vi "ROS_Topic_Close.vi"(0 "error in":errorcluster, 2 "topic":string, 3 "StopConsole":bool=TRUE) -> (1 "error out":errorcluster)   [LabVIEW 2012]
doc: "Closes a topic. If no topic is defined, it will close all tasks and close the console (unless specified otherwise)."
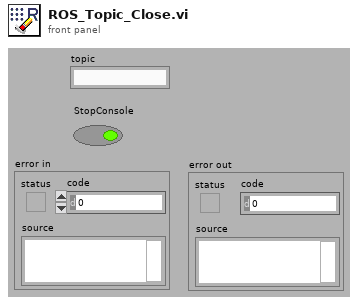
[diagram p1: front panel]
types:
  T1 = enum16{"Add Server", "Clear Server", "Clear All", "Get Info"}
  T2 = typedef "ServoInfo.ctl" = cluster{"vi name":string, "VI Refnum":refnum<vi>, "queue":refnum<queue>, "ROS":T3, "notifier":refnum<notifier>}
  T3 = typedef "_ROSControl.ctl" = cluster{"topic port":u16, "Node":string, "topic":string, "type":string, "node port":u16, "error ":errorcluster, "Direction":T4, "APIs":string[], "Update (ms)":u16, "write queue":u16}
  T4 = typedef "_ROSDirection.ctl" = enum16{"Node", "Publisher", "Subscriber", "Service Client"}
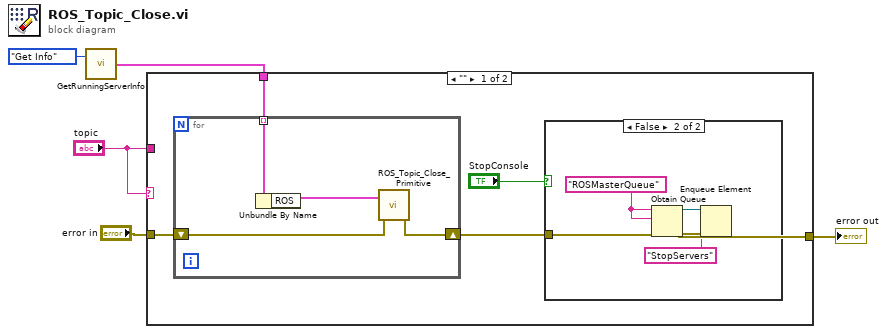
[diagram p0: block diagram]
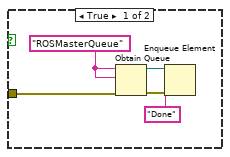
[diagram p2: hidden frame]
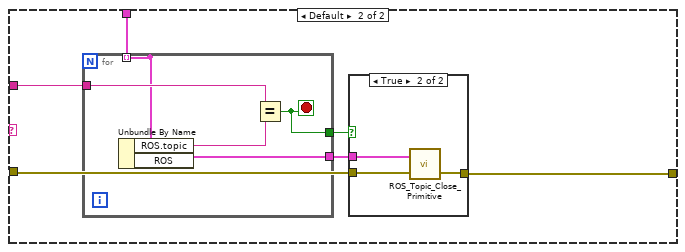
[diagram p3: hidden frame]
diagram:
  n1 = call <userlib>:"GetRunningServerInfo.vi"("Task"=T1."Get Info") -> ("servers"=w1:T2[])  [unwired: 1 in, 2 out]
  n2 = case shown="\"\"" "topic" {
    tunnel: "topic" -> [_ w28]
    tunnel: [w8 w27] -> w5
    tunnel: "error in" -> [w7 w26]
    tunnel: w1 -> [w6 w25]
    frame "" {
      n3 = for {
        shift-right: [w22] -> w8
        shift-left: w7 -> [w23]
        tunnel: w6 -> [w21] mode=indexing
        n4 = Unbundle By Name(w21) -> ("ROS"=w20:T3)
        n5 = call <userlib>:"ROS_Topic_Close_Primitive.vi"("error in"=w23, "ROS in"=w20) -> ("error out"=w22:errorcluster)  [unwired: 1 in]
      }
      n6 = case shown="False" "StopConsole" {
        tunnel: w8 -> [w11 w16]
        frame True {
          w13 = "ROSMasterQueue" ("name (unnamed)")
          n7 = Obtain Queue(name (unnamed)=w13, element data type=w13, error in (no error)=w11) -> (queue out=w14:refnum<queue>, error out=w10:errorcluster)  [unwired: 2 in, 1 out]
          n8 = Enqueue Element(queue=w14, element="Done", error in (no error)=w10) -> ()  [unwired: 1 in, 3 out]
        }
        frame False {
          w18 = "ROSMasterQueue" ("name (unnamed)")
          n9 = Obtain Queue(name (unnamed)=w18, element data type=w18, error in (no error)=w16) -> (queue out=w19:refnum<queue>, error out=w15:errorcluster)  [unwired: 2 in, 1 out]
          n10 = Enqueue Element(queue=w19, element="StopServers", error in (no error)=w15) -> ()  [unwired: 1 in, 3 out]
        }
      }
    }
    frame Default {
      n11 = for {
        tunnel: w28 -> [w38]
        tunnel: [w37] -> w29
        tunnel: [w36] -> _ mode=indexing
        tunnel: w25 -> [w36] mode=indexing
        tunnel: [w35] -> w24
        stop <- w37 stop-if-true
        n12 = Unbundle By Name(w36) -> ("ROS.topic"=w34:string, "ROS"=w35:T3)
        n13 = Equal?(x=w38, y=w34) -> (x = y?=w37:bool)
      }
      n14 = case shown="True" w29 {
        tunnel: [w30 w33] -> w27
        tunnel: w26 -> [w30 w32]
        tunnel: w24 -> [_ w31]
        frame False {
        }
        frame True {
          n15 = call <userlib>:"ROS_Topic_Close_Primitive.vi"("error in"=w32, "ROS in"=w31) -> ("error out"=w33:errorcluster)  [unwired: 1 in]
        }
      }
    }
  }
  "error out" <- w5
